vi "Set Remote Mode.vi"(8 "error in (no error)":errorcluster, 11 ".NET Refnum in":refnum<k24>) -> (0 "error out":errorcluster, 3 ".NET Refnum out":refnum<k24>)   [LabVIEW 2019, in "ESP301-Driver.lvlib"]
uses:
  ESP301-Driver.lvlib
  Newport.ESP301.CommandInterface
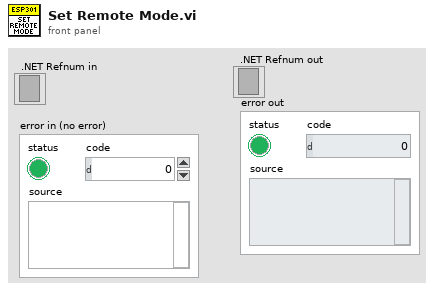
[diagram p1: front panel]
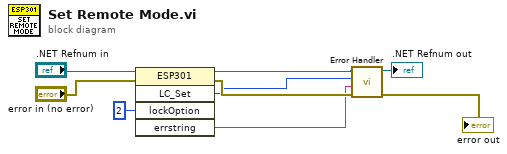
[diagram p0: block diagram]
diagram:
  n1 = invoke class="ESP301" method="LC_Set"(reference=".NET Refnum in", error in="error in (no error)", "lockOption"=2) -> (reference out=w6:refnum<k24>, error out=w5:errorcluster, "LC_Set"=w3:i32, "errstring"=w4:string)  [unwired: 2 in, 1 out]
  n2 = call "Error Handler.vi"("error in (no error)"=w5, "Message"=w4, "Error Code"=w3, ".NET Refnum in"=w6) -> ("error out"=→"error out":errorcluster, ".NET Refnum out"=→".NET Refnum out":refnum<k24>)  [unwired: 6 in]
